vi "Simple PWM.vi"(8 "Compare Value":u16, 11 "PWM":refnum<k21>) -> ()   [LabVIEW 2018]
uses:
  <vilib>/rvi/eio/common/nirviEmuTemplateMethod_errors.vi
  <vilib>/eio/EIONode/EIONode.xnode
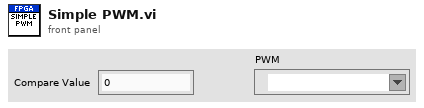
[diagram p1: front panel]
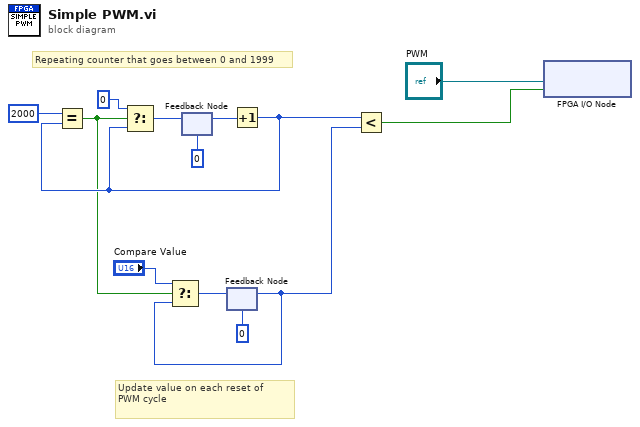
[diagram p0: block diagram]
diagram:
  # "Repeating counter that goes between 0 and 1999"
  # "Update value on each reset of \nPWM cycle"
  n1 = feedback #1(u16 0 ("Compare Value")) -> (w8:u16)
  n2 = feedback #2(u16 0 ("Compare Value")) -> (w4:u16)
  n3 = Increment(x=w8) -> (x+1=w5:u16)
  n4 = Equal?(x=u16 2000 ("Compare Value"), y=w5) -> (x = y?=w3:bool)
  n5 = Select(t=u16 0, s=w3, f=w5) -> (s? t:f=w10:u16)
  n6 = Select(t="Compare Value", s=w3, f=w4) -> (s? t:f=w12:u16)
  n7 = feedback-in #1(w10) -> ()
  n8 = feedback-in #2(w12) -> ()
  n9 = Less?(x=w5, y=w4) -> (x < y?=w1:bool)
  n10 = xnode "FPGA I/O Node"("I/O Item"=w1, "FPGA I/O In"="PWM") -> ()  [unwired: 1 out]
